vi "GetExtReferenceClockFrequency.vi"(3 "error in (no error)":errorcluster, 4 "Return Parameter":u8(ring) items=["Frequency Value", "Minimum", "Maximum"], 5 "VISA resource name":refnum<visa-resource-name>) -> (0 "error out":errorcluster, 1 "External Reference Clock (Hz)":dbl format="%#_16g", 2 "VISA resource name out":refnum<visa-resource-name>)   [LabVIEW 2020, in "Active Technologies AWG3000.lvlib"]
uses:
  Active Technologies AWG3000.lvlib
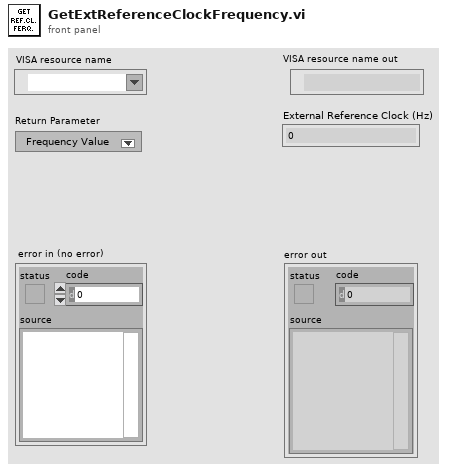
[diagram p1: front panel]
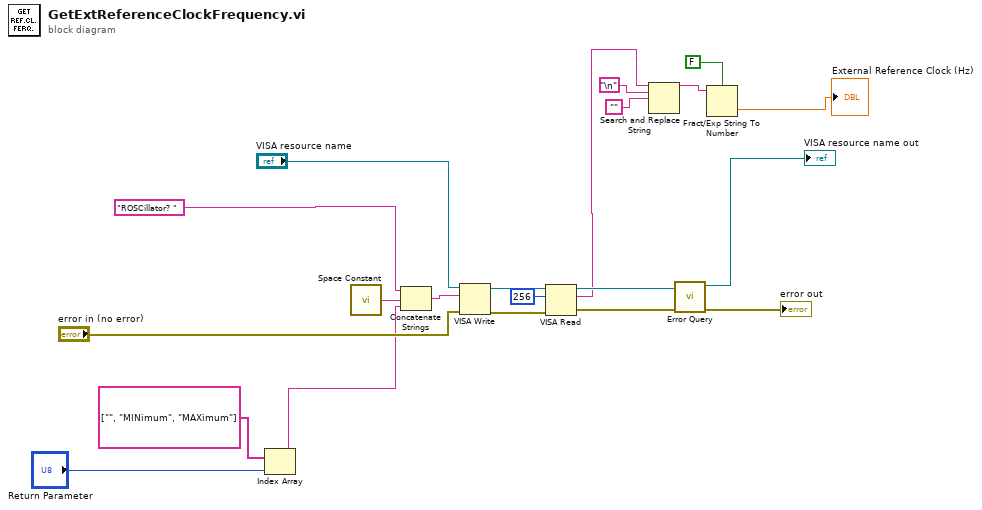
[diagram p0: block diagram]
diagram:
  n1 = Index Array(array=string[] ["", "MINimum", "MAXimum"], index="Return Parameter") -> (element=w10:string)
  n2 = call <vilib>:"Space Constant.vi"() -> ("String"=w9:string)
  n3 = Concatenate Strings("ROSCillator? " ("write buffer"), w9, w10) -> (w8:string)
  n4 = VISA Write(VISA resource name="VISA resource name", write buffer=w8, error in (no error)="error in (no error)") -> (VISA resource name out=w19:refnum<visa-resource-name>, error out=w18:errorcluster)  [unwired: 1 out]
  n5 = VISA Read(VISA resource name=w19, byte count=u32 256, error in (no error)=w18) -> (VISA resource name out=w16:refnum<visa-resource-name>, read buffer=w3:string, error out=w15:errorcluster)  [unwired: 1 out]
  n6 = Search and Replace String(input string=w3, search string="\n", replace string="") -> (result string=w5:string)  [unwired: 5 in, 3 out]
  n7 = call "Error Query.vi"("error in (no error)"=w15, "VISA resource name"=w16) -> ("error out"=→"error out":errorcluster, "VISA resource name out"=→"VISA resource name out":refnum<visa-resource-name>)  [unwired: 6 in, 2 out]
  n8 = Fract/Exp String To Number(use system decimal point (T)=FALSE, string=w5) -> (number=→"External Reference Clock (Hz)":dbl)  [unwired: 2 in, 1 out]
